vi "weight set param.vi"(10 "Q3":dbl caption="mg/s" format="%#.0f", 11 "PV weight":dbl caption="g" format="%#.0f") -> (2 "Q 1":dbl caption="mg/s" format="%#.0f", 3 "Weight 1":dbl caption="g" format="%#.0f")   [LabVIEW 2019]
panel:
  in  "Tab Control":T1(tab)
  out "dM 3":dbl caption="g" format="%#.0f"
  out "dM 1":dbl caption="g" format="%#.0f"
  in  "Tare":dbl caption="g" format="%#.0f"
  in  "<0>":bool
  in  "<вес>":bool
  in  "k":dbl=1.0 caption="g" format="%#.3f"
  in  "Вес":dbl caption="g" format="%#.0f"
  # "Усреднение за 1 мин"
  # "(расход)"
  # "Усреднение за 3 мин"
  # "(расход)"
  # "Вес тары\n(полностью очистить бункер от продукта\nи запомнить PV weight или ввести вручную)."
  # "Вес тары\n(ввести фактический вес без учета тары\nили ввести k вручную)"
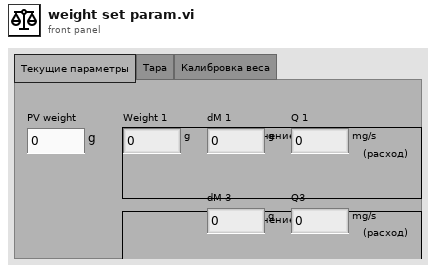
[diagram p1: front panel]
types:
  T1 = enum32{"Текущие параметры", "Тара", "Калибровка веса"}
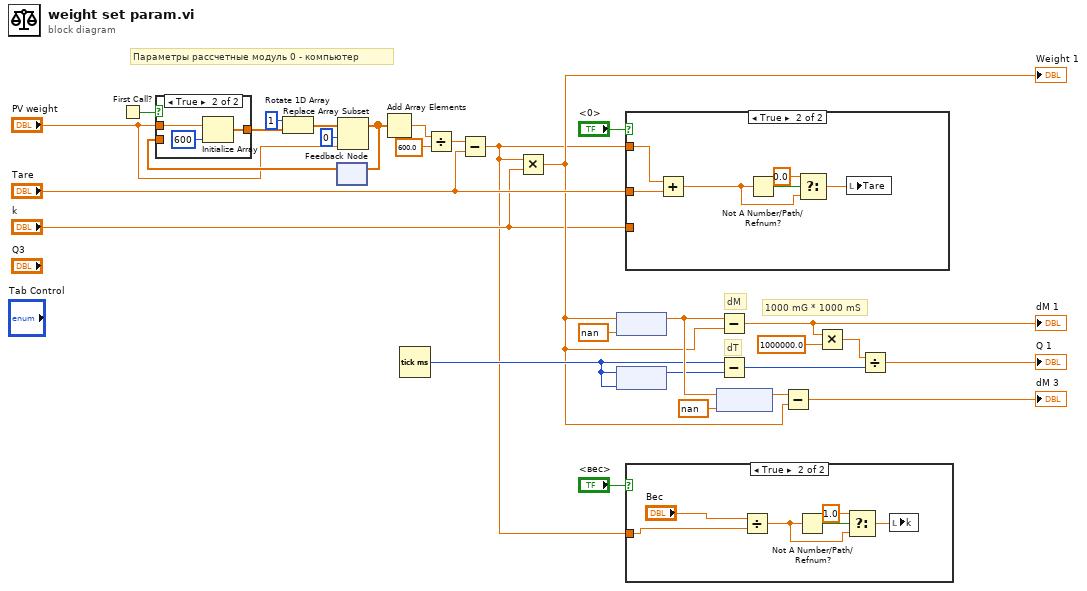
[diagram p0: block diagram]
diagram:
  # "1000 mG * 1000 mS"
  # "dM"
  # "dT"
  # "Параметры рассчетные модуль 0 - компьютер"
  n1 = First Call?() -> (First Call?: T/F=w22:bool)
  n2 = feedback #1() -> (w24:dbl[])  [unwired: 1 in]
  n3 = case shown="True" w22 {
    tunnel: [w30 w32] -> w23
    tunnel: "PV weight" -> [_ w31]
    tunnel: w24 -> [w30 _]
    frame False {
    }
    frame True {
      n4 = Initialize Array(w31, 600 ("dimension size")) -> (w32:dbl[])
    }
  }
  n5 = Rotate 1D Array(1:w23, 2:1 ("n")) -> (0:w28:dbl[])
  n6 = Replace Array Subset(array=w28, new element="PV weight", index=0) -> (w3:dbl[])
  n7 = feedback-in #1(w3) -> ()
  n8 = Add Array Elements(numeric array=w3) -> (sum=w25:dbl)
  n9 = Tick Count (ms)() -> (millisecond timer value=w13:u32)
  n10 = Divide(x=w25, y=600.0) -> (x/y=w1:dbl)
  n11 = Subtract(x=w1, y="Tare") -> (x-y=w4:dbl)
  n12 = Multiply(x=w4, y="k") -> (x*y=w6:dbl)
  "Weight 1" <- w6
  n13 = feedback #2(nan) -> (w17:dbl)
  n14 = feedback-in #2(w6) -> ()
  n15 = feedback #3(w13) -> (w12:u32)
  n16 = feedback-in #3(w13) -> ()
  n17 = case shown="True" "<0>" {
    tunnel: "Tare" -> [_ w36]
    tunnel: w4 -> [_ w35]
    tunnel: "k" -> [_ _]
    frame False {
    }
    frame True {
      n18 = Add(x=w35, y=w36) -> (x+y=w34:dbl)
      n19 = Not A Number/Path/Refnum?(number/path/refnum=w34) -> (NaN/Path/Refnum?=w39:bool)
      n20 = Select(t=0.0 ("y"), s=w39, f=w34) -> (s? t:f=w37:dbl)
      n21 = local write "Tare"(w37) -> ()
    }
  }
  n22 = case shown="True" "<вес>" {
    tunnel: w4 -> [_ w40]
    frame False {
    }
    frame True {
      n23 = Divide(x="Вес", y=w40) -> (x/y=w43:dbl)
      n24 = Not A Number/Path/Refnum?(number/path/refnum=w43) -> (NaN/Path/Refnum?=w45:bool)
      n25 = Select(t=1.0 ("y"), s=w45, f=w43) -> (s? t:f=w42:dbl)
      n26 = local write "k"(w42) -> ()
    }
  }
  n27 = feedback #4(nan) -> (w18:dbl)
  n28 = feedback-in #4(w17) -> ()
  n29 = Subtract(x=w17, y=w6) -> (x-y=w10:dbl)
  "dM 1" <- w10
  n30 = Subtract(x=w13, y=w12) -> (x-y=w8:u32)
  n31 = Subtract(x=w18, y=w6) -> (x-y=→"dM 3":dbl)
  n32 = Multiply(x=w10, y=1000000.0) -> (x*y=w9:dbl)
  n33 = Divide(x=w9, y=w8) -> (x/y=→"Q 1":dbl)
